vi "CheckboxList.vi"() -> ()   [LabVIEW 2021]
uses:
  System.Windows.Forms
panel:
  out "error out":errorcluster
  in  "NbCheckBoxes":i32=20
  out "Selection":string[](array[string])
  in  "CheckedListBox":refnum<k24>(container)
  in  "stop":bool
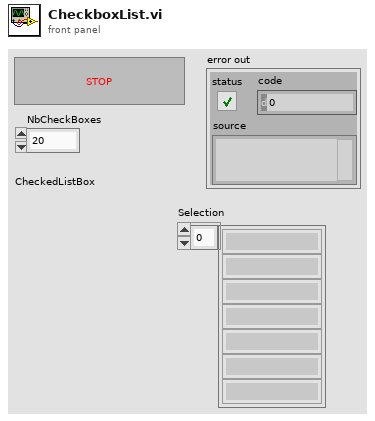
[diagram p1: front panel]
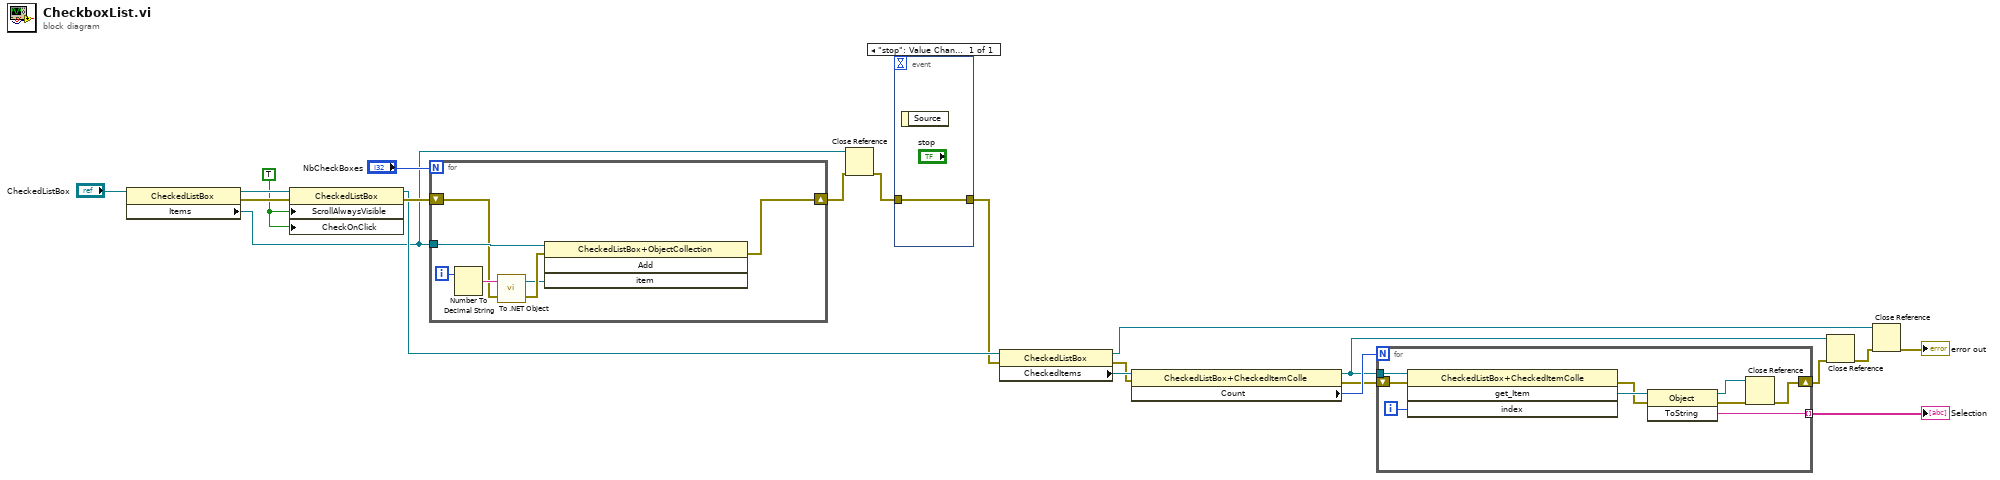
[diagram p0: block diagram]
diagram:
  w16 = TRUE ("ScrollAlwaysVisible")
  n1 = property class="CheckedListBox"(reference="CheckedListBox") -> (reference out=w20:refnum<k24>, error out=w18:errorcluster, "Items"=w9:refnum<k24>)  [unwired: 1 in]
  n2 = property class="CheckedListBox"(reference=w20, error in=w18, "ScrollAlwaysVisible"=w16, "CheckOnClick"=w16) -> (reference out=w15:refnum<k24>, error out=w17:errorcluster)
  n3 = for {
    N: "NbCheckBoxes" -> [_]
    tunnel: w9 -> [w28]
    shift-right: [w27] -> w8
    shift-left: w17 -> [w24]
    i -> [w25]
    n4 = Number To Decimal String(number=w25) -> (decimal integer string=w26:string)  [unwired: 1 in]
    n5 = call <vilib>:"To .NET Object.vi"("error in (no error)"=w24, "anything"=w26) -> ("error out"=w23:errorcluster, ".NET object"=w22:refnum<k24>)
    n6 = invoke class="CheckedListBox+ObjectCollection" method="Add"(reference=w28, error in=w23, "item"=w22) -> (error out=w27:errorcluster)  [unwired: 1 in, 3 out]
  }
  n7 = Close Reference(reference=w9, error in (no error)=w8) -> (error out=w7:errorcluster)
  n8 = event shown="[0] \"stop\": Value Change" {
    selector: _ -> [_]
    dyn-events: _ -> [_]
    timeout: _ -> [_]
    tunnel: w7 -> [w29]
    tunnel: [w29] -> w6
    event "stop": Value Change {
      n9 = event-data() -> ()  [unwired: 1 in, 1 out]
    }
  }
  n10 = property class="CheckedListBox"(reference=w15, error in=w6) -> (reference out=w3:refnum<k24>, error out=w11:errorcluster, "CheckedItems"=w14:refnum<k24>)
  n11 = property class="CheckedListBox+CheckedItemColle"(reference=w14, error in=w11) -> (reference out=w5:refnum<k24>, error out=w10:errorcluster, "Count"=w13:i32)
  n12 = for {
    N: w13 -> [_]
    tunnel: w5 -> [w38]
    tunnel: [w35] -> w12 mode=indexing
    shift-right: [w30] -> w4
    shift-left: w10 -> [w34]
    i -> [w37]
    n13 = invoke class="CheckedListBox+CheckedItemColle" method="get_Item"(reference=w38, error in=w34, "index"=w37) -> (error out=w33:errorcluster, "get_Item"=w36:refnum<k24>)  [unwired: 1 in, 2 out]
    n14 = invoke class="Object" method="ToString"(reference=w36, error in=w33) -> (reference out=w32:refnum<k24>, error out=w31:errorcluster, "ToString"=w35:string)  [unwired: 1 in]
    n15 = Close Reference(reference=w32, error in (no error)=w31) -> (error out=w30:errorcluster)
  }
  "Selection" <- w12
  n16 = Close Reference(reference=w5, error in (no error)=w4) -> (error out=w2:errorcluster)
  n17 = Close Reference(reference=w3, error in (no error)=w2) -> (error out=→"error out":errorcluster)
